vi "Text control_KM.vi"() -> ()   [LabVIEW 2016]
panel:
  in  "Panel Controls 2":T1={"Emergency Stop"=refnum, "TransGraph Max"=1e-05, "Text/Graph (text=false)"=FALSE, "TransGraph Min"=1e-11} {"TransGraph Min" format="%.2e"; "TransGraph Max" format="%.2e"}
  out "Currently running:":string
  in  "Lines left to run:":string
  in  "Standby":T2
  in  "Full Reset":bool
  in  "SMU4":cluster{"on/off":bool, "Voltage":dbl} {"Voltage" min=-100.0 max=100.0 format="%.2f"}
  in  "Source/Drain\nRange":u8(slide)=6 max=11 scale=0.0..11.0
  in  "Source/Drain\nRange mode":u16(ring) items=["Auto", "Limited", "Fixed"]
  in  "Gate Range":u8(slide)=6 max=11 scale=0.0..11.0
  in  "Gate Range\nmode":u16(ring) items=["Auto", "Limited", "Fixed"]
  in  "Gate":T3={"Gate Start"=0.0, "Gate Stop"=2.0, "Gate Step (linear only)"=1.0, "Gate Compliance"=0.0001, "Gate PComp"=0.0, "Range mode"=0, "Range"=6} {"Range" max=11 scale=0.0..11.0; "Range mode" items=["Auto", "Limited", "Fixed"]; "Gate PComp" format="%^.2e"; "Gate Compliance" format="%^.2e"; "Gate Step (linear only)" format="%^.4e"; "Gate Stop" format="%^.4e"; "Gate Start" format="%^.4e"}
  in  "Drain 2":T4={"Drain Start"=0.0, "Drain Stop"=2.0, "Drain Compliance"=0.0001, "Drain Step"=1.0, "Drain PComp"=0.0, "Range mode"=0, "Range"=6} {"Range" max=11 scale=0.0..11.0; "Range mode" items=["Auto", "Limited", "Fixed"]; "Drain PComp" format="%^.2e"; "Drain Step" format="%^.4e"; "Drain Compliance" format="%^.2e"; "Drain Stop" format="%^.4e"; "Drain Start" format="%^.4e"}
  in  "Timings 2":T5={"integration time"=0, "Short/Long integration time"=0.00064, "hold time (sec)"=0.0, "delay time (sec)"=0.0, "Step Time (0 disables)"=0.0, "sweep method"=0, "Pulse period"=0.005, "Base voltage"=0.0, "Pulse width"=0.0005} {"Pulse width" min=0.0005 max=0.1 step=0.0001 format="%.4f"; "Base voltage" format="%^.4e"; "Pulse period" min=0.005 max=1.0 step=0.0001 format="%.4f"; "sweep method" items=["Continuous", "Pulsed"]; "Step Time (0 disables)" format="%.2f"; "delay time (sec)" format="%.4f"; "hold time (sec)" format="%.4f"; "Short/Long integration time" format="%^.0e"; "integration time" scale=0.0..2.0}
  in  "Panel Controls":T6={"Emergency Stop"=refnum, "TransGraph Max"=1e-05, "Text/Graph (text=false)"=TRUE} {"TransGraph Max" format="%.2e"}
  in  "Interrupt run":bool
  in  "Drain: Compliance":dbl=0.001 format="%.8f"
  in  "Gate: Compliance":dbl=0.001 format="%.8f"
  out "Path":path
  in  "hold time /s":dbl format="%.2f"
  in  "delay time /s":dbl format="%.2f"
  in  "integration time":u32(slide)=1 max=2 step=1 scale=0.0..2.0
  in  "Integration time (short)":dbl=0.0019 min=8e-05 max=0.0019 step=8e-05 format="%^.0e"
  in  "Integration time (long)":dbl=0.32 min=0.04 max=2.0 step=0.02 format="%.2f"
  in  "Step delay /s":dbl format="%.2f"
  in  "Program":string="sample -60 -5 100 240\ntransfer d 10 -60 -1 -5 -60 -55"
  # "Syntax:\nsample Vg Vd NumSamples Time\nwait NumMilliseconds\nwait-min NumMinutes\ntransfer [s|d] VgStart VgStop VgStep VdStart VdStop VdStep\noutput [s|d] VgStart VgStop VgStep VdStart VdStop VdStep\nitime [s|m|l]\ngaterangemode [a|l|f]\ndrainrangemode [a|l|f]\nstandby [on l off]\nsample-fpp Vg Vd NumSamples Time\nresample-fpp Vg Vd\ntransfer-fpp [s|d] VgStart VgStop VgStep VdStart VdStop VdStep\noutput-fpp [s|d] VgStart VgStop VgStep VdStart VdStop VdStep"
  # "100 samples is approx 13s with medium integration"
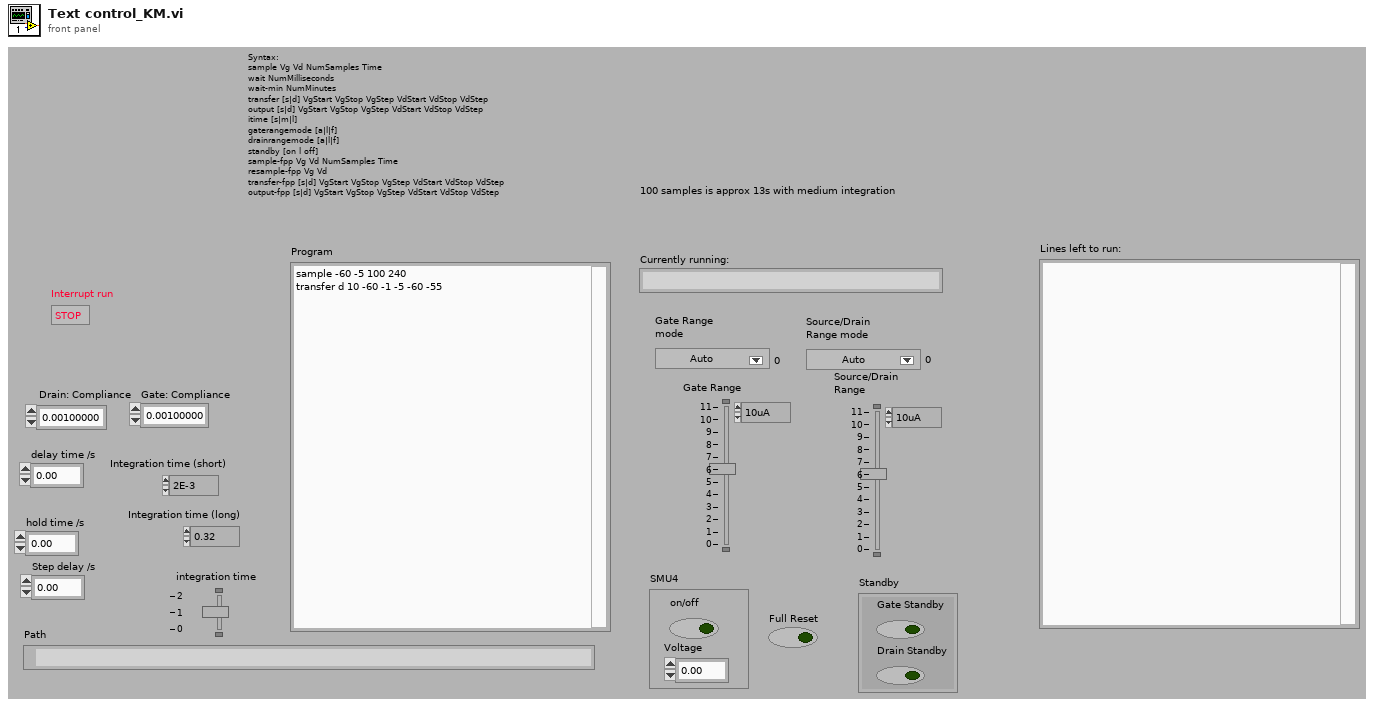
[diagram p1: front panel]
types:
  T1 = cluster{"Emergency Stop":refnum<vi>, "TransGraph Max":dbl, "Text/Graph (text=false)":bool, "TransGraph Min":dbl}
  T2 = cluster{"Gate Standby":bool, "Drain Standby":bool}
  T3 = cluster{"Gate Start":dbl, "Gate Stop":dbl, "Gate Step (linear only)":dbl, "Gate Compliance":dbl, "Gate PComp":dbl, "Range mode":u16, "Range":u8}
  T4 = cluster{"Drain Start":dbl, "Drain Stop":dbl, "Drain Compliance":dbl, "Drain Step":dbl, "Drain PComp":dbl, "Range mode":u16, "Range":u8}
  T5 = cluster{"integration time":u32, "Short/Long integration time":dbl, "hold time (sec)":dbl, "delay time (sec)":dbl, "Step Time (0 disables)":dbl, "sweep method":u16, "Pulse period":dbl, "Base voltage":dbl, "Pulse width":dbl}
  T6 = cluster{"Emergency Stop":refnum<vi>, "TransGraph Max":dbl, "Text/Graph (text=false)":bool}
  T7 = enum16{"open", "replace", "create", "open or create", "replace or create", "replace or create with confirmation"}
  T8 = cluster{"V2 Start":dbl, "V2 Step":dbl, "Number of points":i32}
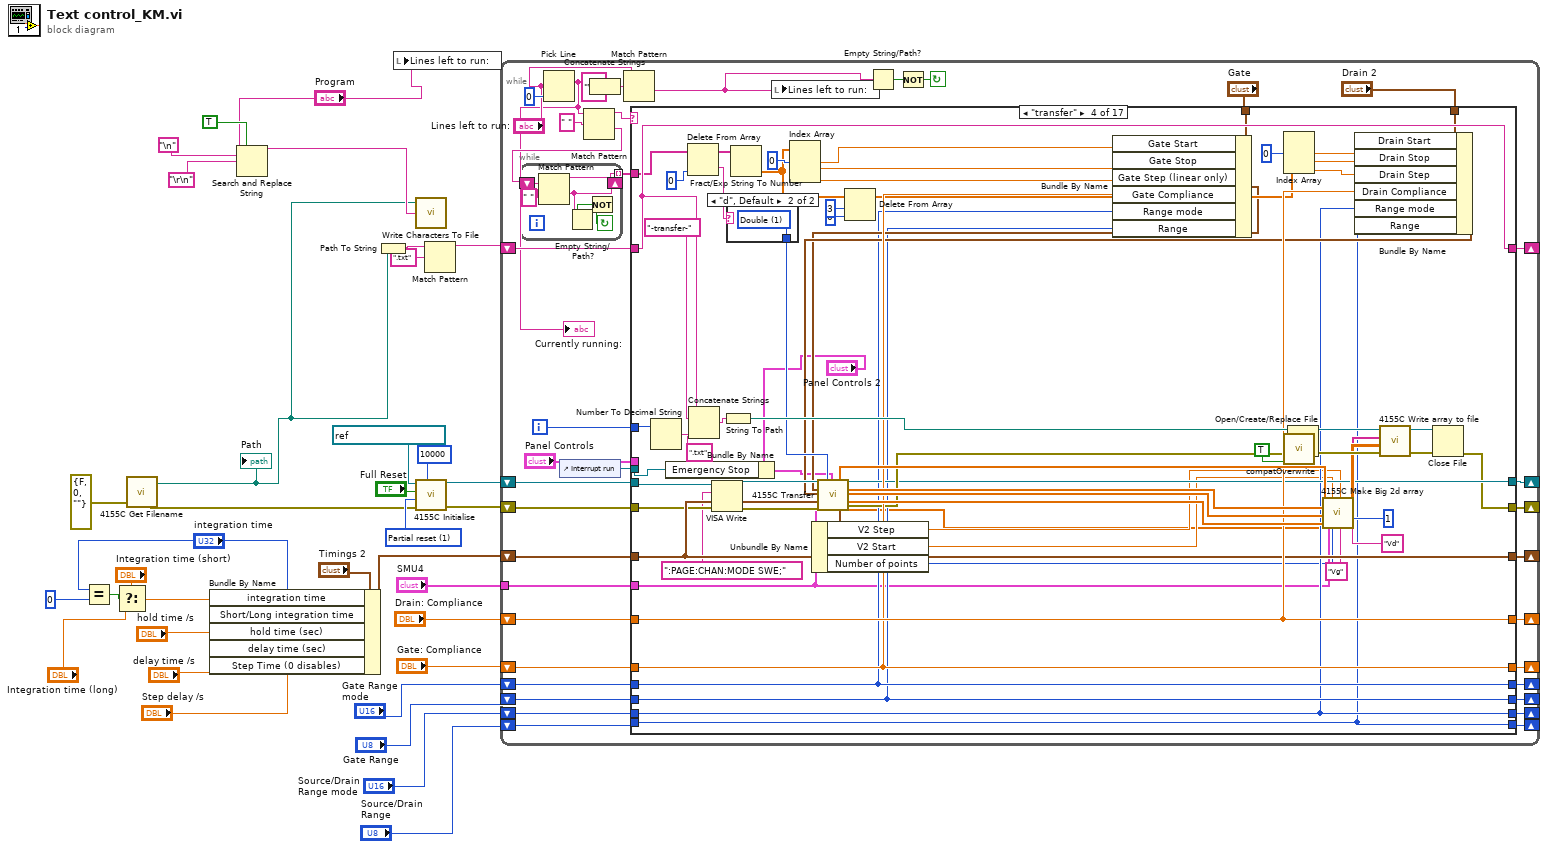
[diagram p0: block diagram]
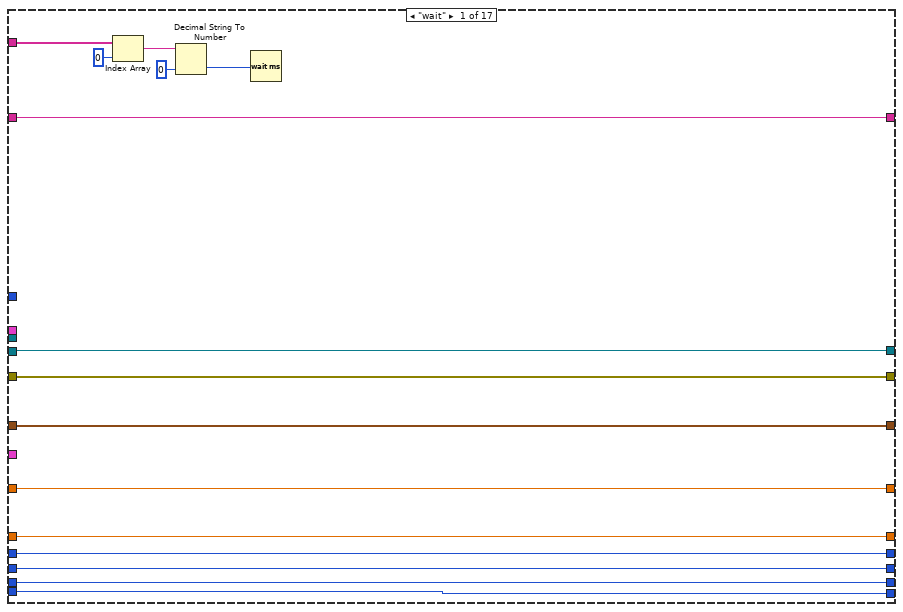
[diagram p2: hidden frame]
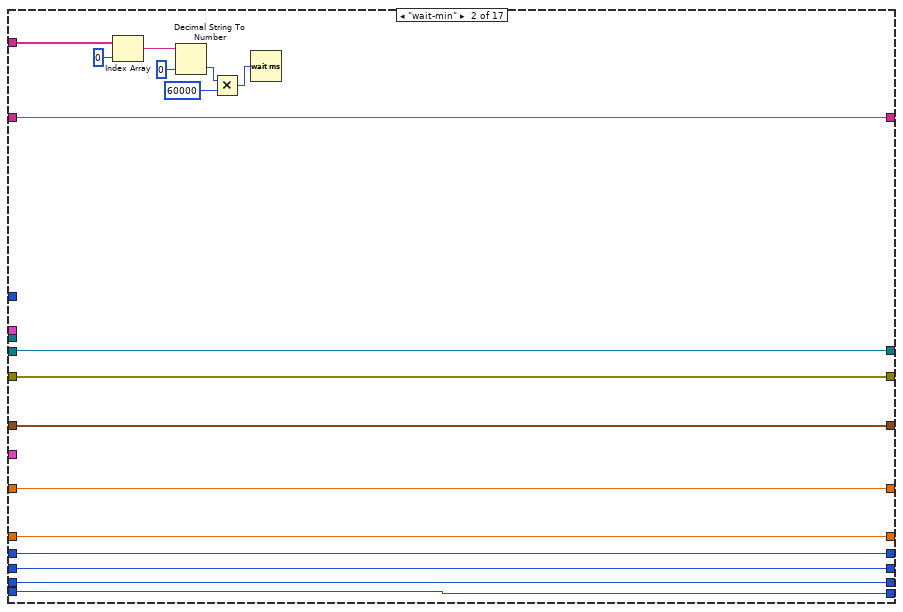
[diagram p3: hidden frame]
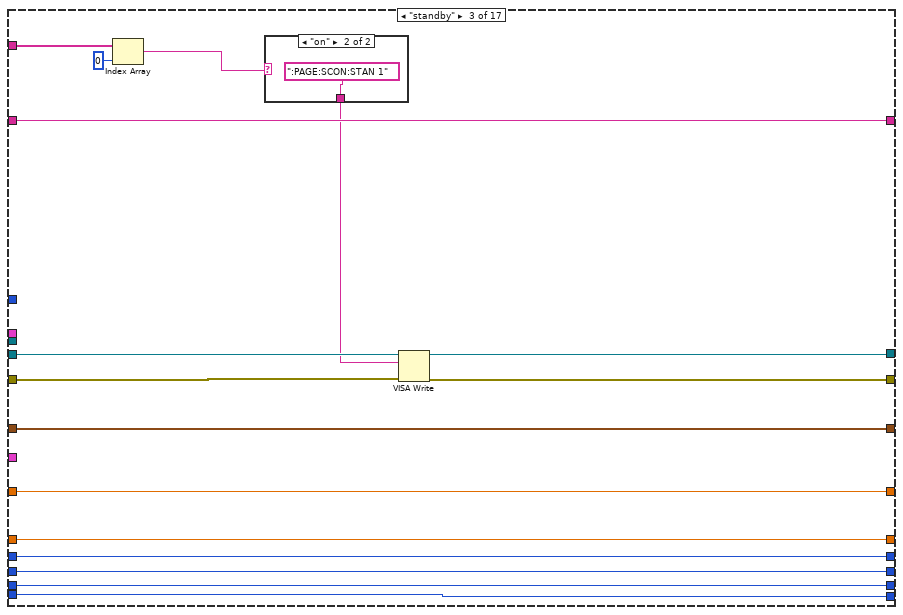
[diagram p4: hidden frame]
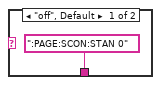
[diagram p5: hidden frame]
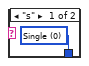
[diagram p6: hidden frame]
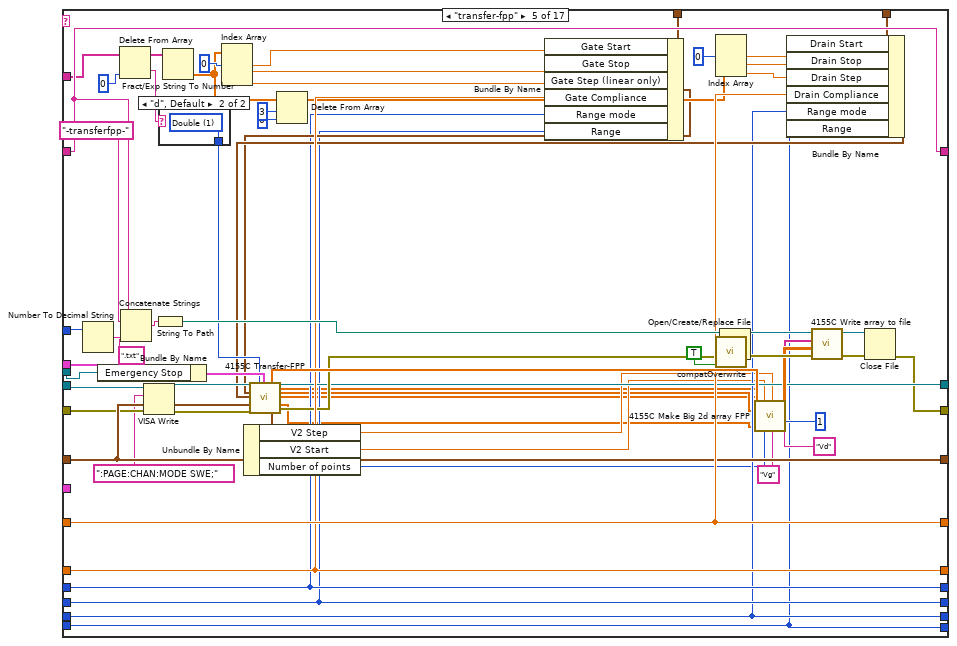
[diagram p7: hidden frame]
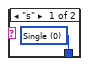
[diagram p8: hidden frame]
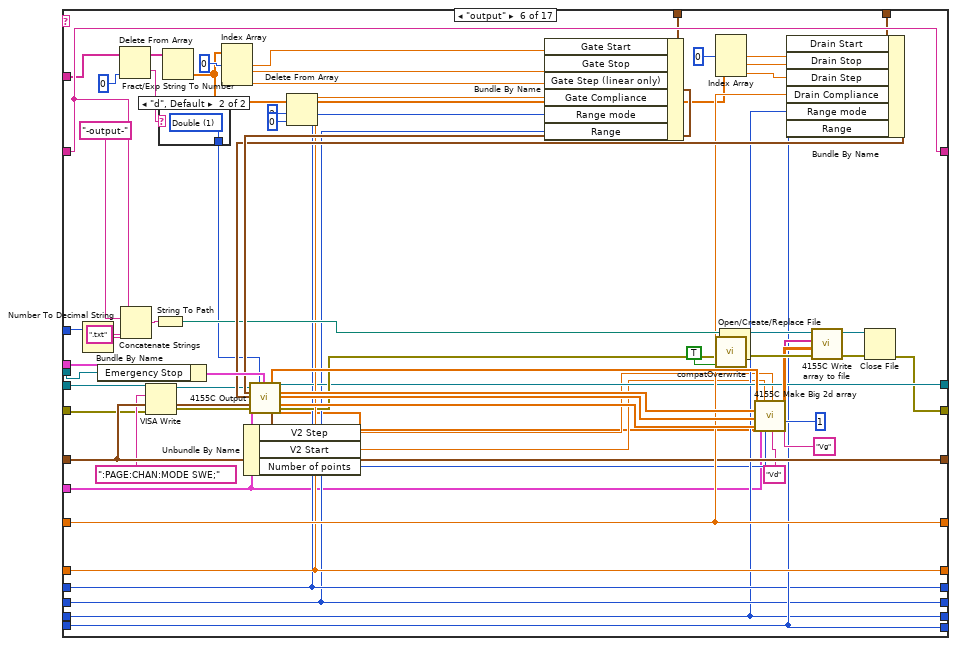
[diagram p9: hidden frame]
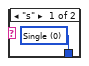
[diagram p10: hidden frame]
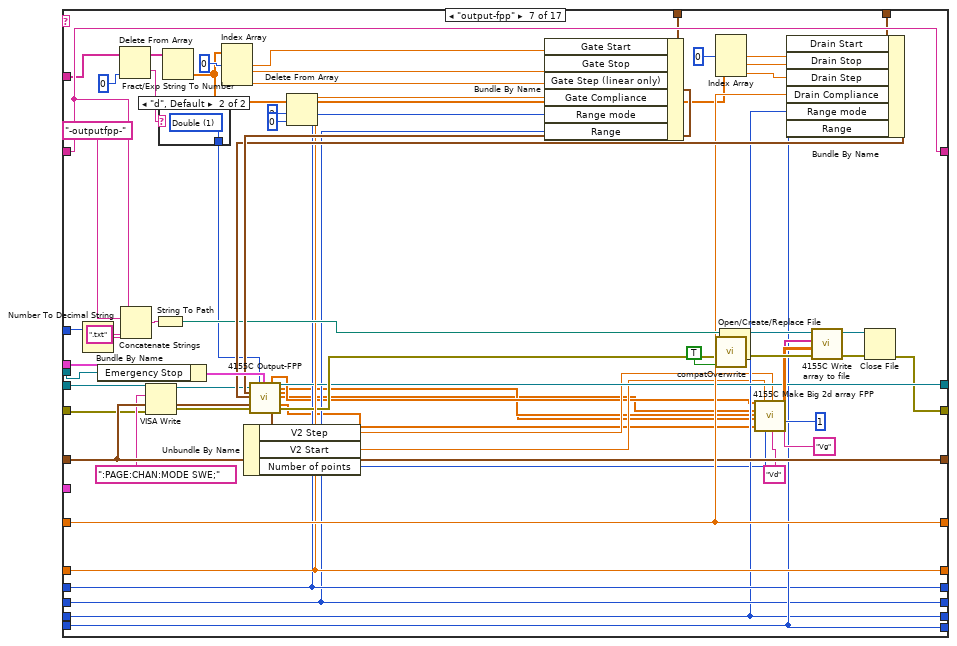
[diagram p11: hidden frame]
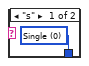
[diagram p12: hidden frame]
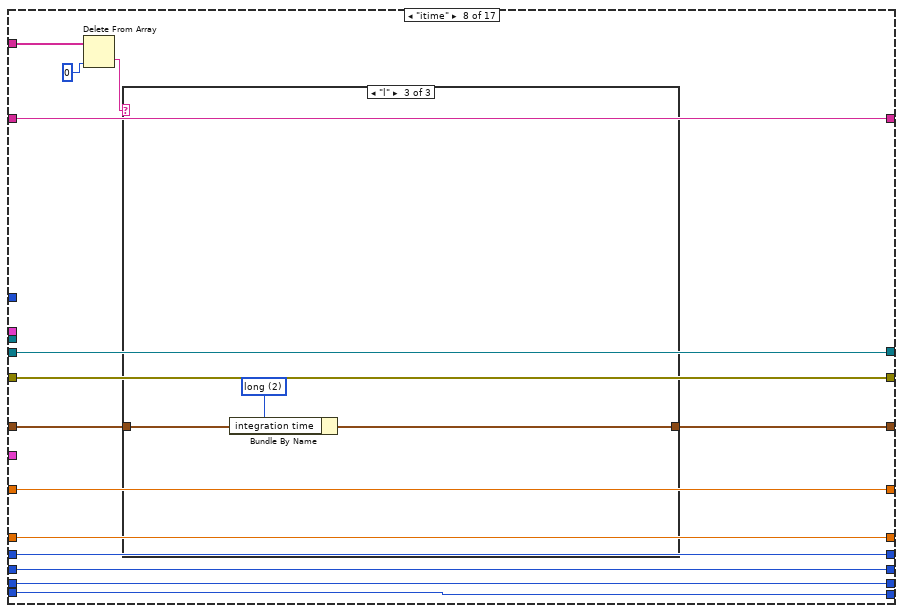
[diagram p13: hidden frame]
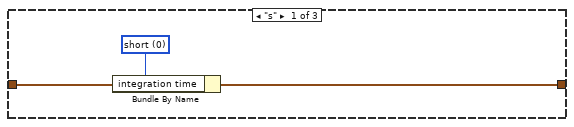
[diagram p14: hidden frame]
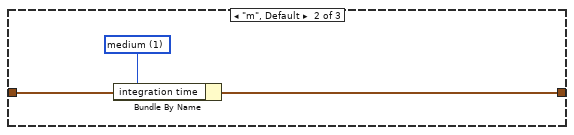
[diagram p15: hidden frame]
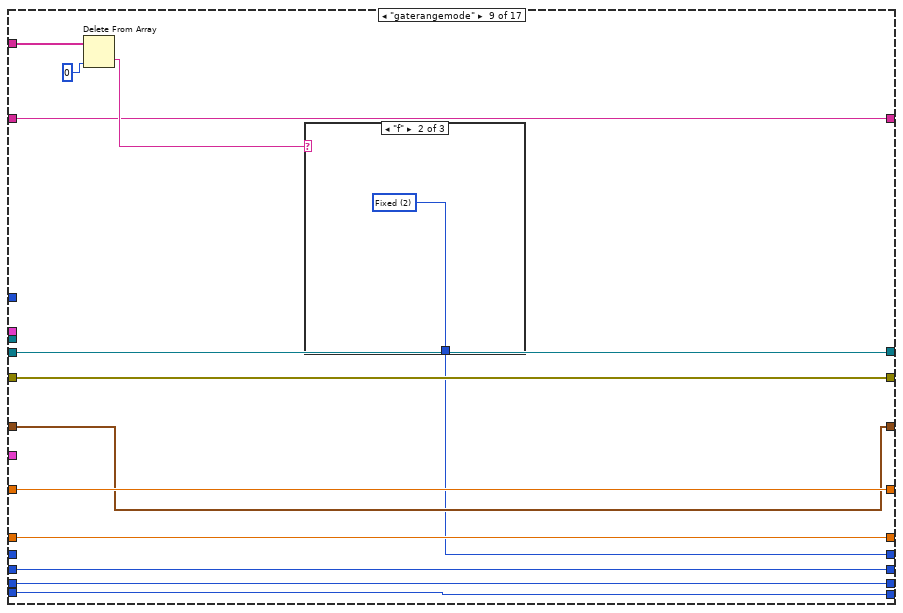
[diagram p16: hidden frame]
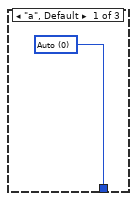
[diagram p17: hidden frame]
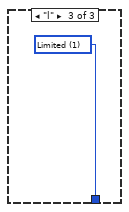
[diagram p18: hidden frame]
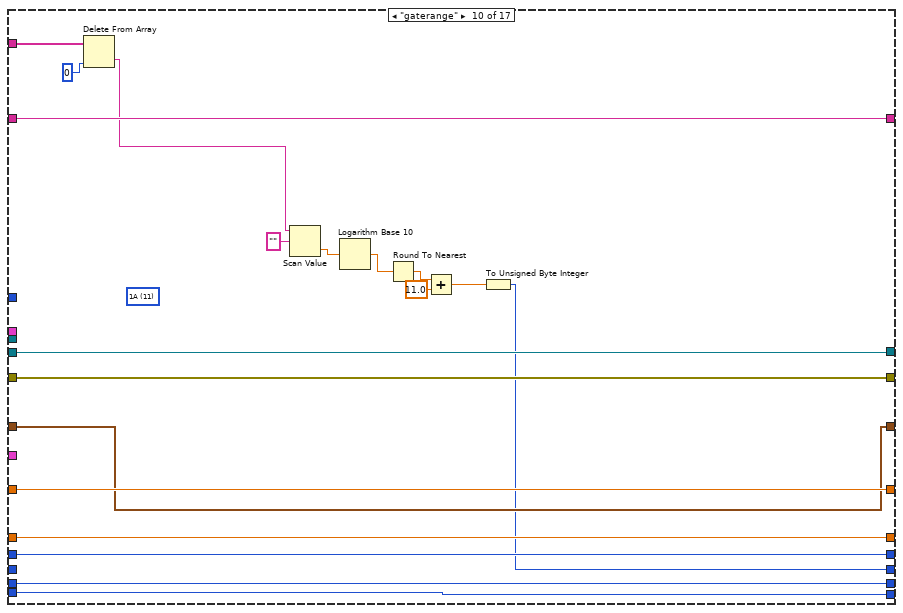
[diagram p19: hidden frame]
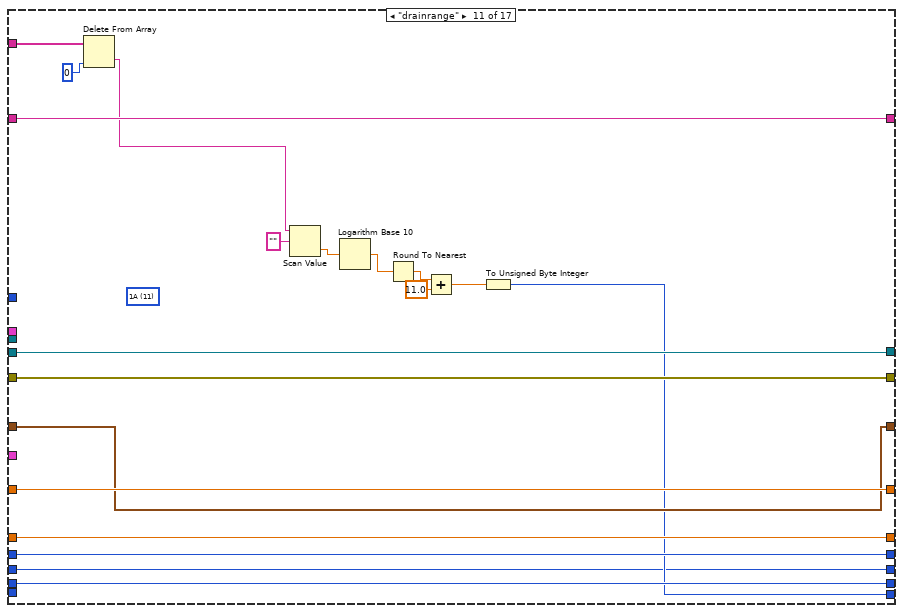
[diagram p20: hidden frame]
diagram:
  w26 = u16 1 items=["Reset All", "Partial reset"] ("Type of reset")
  n1 = Equal?(x="integration time", y=u32 0) -> (x = y?=w30:bool)
  n2 = Select(t="Integration time (short)", s=w30, f="Integration time (long)") -> (s? t:f=w34:dbl)
  n3 = call "4155C Get Filename.vi"("error in (no error)"=errorcluster {"status"=FALSE, "code"=0, "source"=""}) -> ("error out"=w21:errorcluster, "path"=w5:path)  [unwired: 2 in, 1 out]
  "Path" <- w5
  n4 = Bundle By Name(cluster="Timings 2", "integration time"="integration time", "Short/Long integration time"=w34, "hold time (sec)"="hold time /s", "delay time (sec)"="delay time /s", "Step Time (0 disables)"="Step delay /s") -> (w18:T5)
  n5 = Search and Replace String(replace all?=TRUE ("replace all? (F)"), input string="Program", search string="\n", replace string="\r\n") -> (result string=w8:string)  [unwired: 4 in, 3 out]
  n6 = Path To String(path=w5) -> (string=w4:string)
  n7 = local write "Lines left to run:"("Program") -> ()
  n8 = call <vilib>:"Write Characters To File.vi"("character string"=w8, "file path (dialog if empty)"=w5) -> ()  [unwired: 3 in, 1 out]
  n9 = call "4155C Initialise.vi"("VISA resource name in"=refnum<visa-resource-name> "GPIB0::14::INSTR", "Reset"="Full Reset", "Type of reset"=w26, "error in (no error)"=w21, "VISA Timeout Value"=u32 10000) -> ("VISA Resource Name out"=w20:refnum<visa-resource-name>, "error out"=w19:errorcluster)
  n10 = Match Pattern(string=w4, regular expression=".txt") -> (before substring=w3:string)  [unwired: 1 in, 3 out]
  n11 = while {
    tunnel: "SMU4" -> [w39]
    shift-left: "Source/Drain\nRange" -> [w44]
    shift-right: [w40] -> _
    shift-left: "Source/Drain\nRange mode" -> [w45]
    shift-right: [w41] -> _
    shift-left: "Gate Range" -> [w46]
    shift-right: [w42] -> _
    shift-left: "Gate Range\nmode" -> [w47]
    shift-right: [w43] -> _
    shift-left: "Gate: Compliance" -> [w59]
    shift-right: [w53] -> _
    shift-left: "Drain: Compliance" -> [w60]
    shift-right: [w54] -> _
    shift-left: w18 -> [w61]
    shift-right: [w55] -> _
    shift-left: w19 -> [w62]
    shift-right: [w56] -> _
    shift-left: w20 -> [w63]
    shift-right: [w57] -> _
    shift-left: w3 -> [w64]
    shift-right: [w52] -> _
    i -> [w58]
    stop <- w72 continue-if-true
    n12 = Pick Line(multi-line string="Lines left to run:", line index=0) -> (output string=w36:string)  [unwired: 1 in]
    "Currently running:" <- w36
    n13 = control-ref of="Interrupt run"() -> (w51:refnum<vi>)
    n14 = Match Pattern(string=w36, regular expression=" ") -> (before substring=w67:string, after substring=w66:string)  [unwired: 1 in, 2 out]
    n15 = while {
      tunnel: [w74] -> w65 mode=indexing
      shift-left: w66 -> [w76]
      shift-right: [w75] -> _
      stop <- w78 continue-if-true
      n16 = Match Pattern(string=w76, regular expression=" ") -> (before substring=w74:string, after substring=w75:string)  [unwired: 1 in, 2 out]
      n17 = Empty String/Path?(string/path=w75) -> (empty?=w79:bool)
      n18 = Not(x=w79) -> (.not. x?=w78:bool)
    }
    n19 = Concatenate Strings(w36, "\n" ("Substring")) -> (w70:string)
    n20 = Match Pattern(string="Lines left to run:", regular expression=w70) -> (after substring=w37:string)  [unwired: 1 in, 3 out]
    n21 = case shown="\"transfer\"" w67 {
      tunnel: w65 -> [w94 w111 w127 w172 w242 w306 w378 w415 w437 w460 w479 w491 _ _ w584 w653 w712]
      tunnel: w64 -> [w89 w107 w125 w180 w250 w314 w386 w404 w429 w453 w473 w484 w501 w539 w562 w647 w708]
      tunnel: w63 -> [w88 w106 w116 w150 w219 w282 w354 w405 w430 w454 w474 w485 w506 w542 w591 w660 w665]
      tunnel: w62 -> [w87 w105 w115 w149 w218 w279 w351 w406 w431 w455 w475 w486 w505 w511 w590 w659 w664]
      tunnel: w61 -> [w86 w104 w124 w176 w246 w310 w382 w414 w428 w452 w472 w483 w504 w535 w553 w646 w707]
      tunnel: w60 -> [w85 w103 w123 w178 w248 w312 w384 w413 w436 w459 w478 w490 w503 w520 w589 w658 w717]
      tunnel: w59 -> [w84 w102 w122 w177 w247 w311 w383 w412 w435 w458 w477 w489 w502 w521 w563 w648 w709]
      tunnel: w58 -> [_ _ _ w181 w251 w315 w387 _ _ _ _ _ _ w537 w588 w657 w716]
      tunnel: [w88 w106 w114 w174 w244 w308 w380 w405 w430 w454 w474 w485 w506 w542 w554 w599 w667] -> w57
      tunnel: [w87 w105 w113 w173 w243 w307 w379 w406 w431 w455 w475 w486 w505 w510 w564 w598 w666] -> w56
      tunnel: [w86 w104 w124 w176 w246 w310 w382 w407 w428 w452 w472 w483 w504 w535 w553 w646 w707] -> w55
      tunnel: [w85 w103 w123 w178 w248 w312 w384 w413 w436 w459 w478 w490 w503 w520 w589 w658 w717] -> w54
      tunnel: [w84 w102 w122 w177 w247 w311 w383 w412 w435 w458 w477 w489 w502 w521 w563 w648 w709] -> w53
      tunnel: [w89 w107 w125 w180 w250 w314 w386 w404 w429 w453 w473 w484 w501 w539 w562 w647 w708] -> w52
      tunnel: w51 -> [_ _ _ w189 w256 w323 w391 _ _ _ _ _ _ _ w559 w618 w683]
      tunnel: "Gate" -> [_ _ _ w159 w229 w293 w365 _ _ _ _ _ _ _ _ _ _]
      tunnel: "Drain 2" -> [_ _ _ w158 w228 w292 w364 _ _ _ _ _ _ _ _ _ _]
      tunnel: "Panel Controls" -> [_ _ _ _ w227 w291 w363 _ _ _ _ _ _ _ _ _ _]
      tunnel: w47 -> [w83 w101 w121 w143 w212 w277 w349 w411 _ w451 w471 w482 w500 w522 w549 w642 w703]
      tunnel: w46 -> [w82 w100 w120 w142 w211 w276 w348 w410 w434 _ w462 w488 w499 w523 w550 w643 w704]
      tunnel: w45 -> [w81 w99 w119 w141 w210 w275 w347 w409 w433 w457 w476 _ w498 w524 w551 w644 w705]
      tunnel: w44 -> [w80 w98 w118 w140 w209 w278 w350 w408 w432 w456 _ w487 w497 w525 w552 w645 w706]
      tunnel: [w83 w101 w121 w143 w212 w277 w349 w411 w427 w451 w471 w482 w500 w522 w549 w642 w703] -> w43
      tunnel: [w82 w100 w120 w142 w211 w276 w348 w410 w434 w443 w462 w488 w499 w523 w550 w643 w704] -> w42
      tunnel: [w81 w99 w119 w141 w210 w275 w347 w409 w433 w457 w476 w481 w498 w524 w551 w644 w705] -> w41
      tunnel: [w80 w98 w118 w140 w209 w278 w350 w408 w432 w456 w463 w487 w497 w525 w552 w645 w706] -> w40
      tunnel: w39 -> [_ _ _ w133 _ w269 _ _ _ _ _ _ _ _ _ _ _]
      frame "wait" {
        n22 = Index Array(array=w94, index=0 ("Index")) -> (element=w92:string)
        n23 = Decimal String To Number(string=w92, default (0L)=u32 0) -> (number=w91:u32)  [unwired: 1 in, 1 out]
        n24 = Wait (ms)(milliseconds to wait=w91) -> ()  [unwired: 1 out]
      }
      frame "wait-min" {
        n25 = Index Array(array=w111, index=0 ("Index")) -> (element=w109:string)
        n26 = Decimal String To Number(string=w109, default (0L)=u32 0) -> (number=w97:u32)  [unwired: 1 in, 1 out]
        n27 = Multiply(x=w97, y=u32 60000) -> (x*y=w96:u32)
        n28 = Wait (ms)(milliseconds to wait=w96) -> ()  [unwired: 1 out]
      }
      frame "standby" {
        n29 = Index Array(array=w127, index=0 ("Index")) -> (element=w117:string)
        n30 = case shown="\"on\"" w117 {
          tunnel: [":PAGE:SCON:STAN 0" ":PAGE:SCON:STAN 1"] -> w112
          frame "off", Default {
          }
          frame "on" {
          }
        }
        n31 = VISA Write(VISA resource name=w116, write buffer=w112, error in (no error)=w115) -> (VISA resource name out=w114:refnum<visa-resource-name>, error out=w113:errorcluster)  [unwired: 1 out]
      }
      frame "transfer" {
        n32 = Number To Decimal String(number=w181) -> (decimal integer string=w182:string)  [unwired: 1 in]
        n33 = Bundle By Name(cluster="Panel Controls 2", "Emergency Stop"=w189) -> (w131:T1)
        n34 = Delete From Array(array=w172, index=0 ("Index")) -> (deleted portion=w170:string, array with subset deleted=w169:string[])  [unwired: 1 in]
        n35 = Concatenate Strings(w180, "-transfer-" ("Substring"), w182, ".txt" ("Substring")) -> (w184:string)
        n36 = VISA Write(VISA resource name=w150, write buffer=":PAGE:CHAN:MODE SWE;" ("write buffer (\"\")"), error in (no error)=w149) -> (VISA resource name out=w147:refnum<visa-resource-name>, error out=w148:errorcluster)  [unwired: 1 out]
        n37 = String To Path(string=w184) -> (path=w179:path)
        n38 = case shown="\"d\", Default" w170 {
          tunnel: [w197 w198] -> w168
          frame "s" {
            w197 = u16 0 items=["Single", "Double"] ("sweep mode")
          }
          frame "d", Default {
            w198 = u16 1 items=["Single", "Double"] ("sweep mode")
          }
        }
        n39 = Fract/Exp String To Number(string=w169) -> (number=w154:dbl[])  [unwired: 3 in, 1 out]
        n40 = Index Array(array=w154, index #1=0 ("Index")) -> (element #1=w167:dbl, element #2=w166:dbl, element #3=w165:dbl)  [unwired: 2 in]
        n41 = Delete From Array(array=w154, length=3 ("Length"), index=0 ("Index")) -> (array with subset deleted=w152:dbl[])  [unwired: 1 out]
        n42 = Bundle By Name(cluster=w159, "Gate Start"=w167, "Gate Stop"=w166, "Gate Step (linear only)"=w165, "Gate Compliance"=w177, "Range mode"=w143, "Range"=w142) -> (w144:T3)
        n43 = Index Array(array=w152, index #1=0 ("Index")) -> (element #1=w162:dbl, element #2=w161:dbl, element #3=w160:dbl)  [unwired: 2 in]
        n44 = call <vilib>:"compatOverwrite.vi"("overwrite (F)"=TRUE) -> ("overwrite?"=w130:T7)
        n45 = Bundle By Name(cluster=w158, "Drain Start"=w162, "Drain Stop"=w161, "Drain Step"=w160, "Drain Compliance"=w178, "Range mode"=w141, "Range"=w140) -> (w145:T4)
        n46 = call "4155C Transfer.vi"("VISA resource name in"=w147, "Gate"=w144, "Drain"=w145, "Timings"=w176, "error in (no error)"=w148, "SMU4"=w133, "sweep mode"=w168, "Panel Controls"=w131) -> ("VG"=w185:dbl[], "Outparams"=w138:T8, "VISA Resource Name out"=w174:refnum<visa-resource-name>, "IS"=w188:dbl[], "ID"=w187:dbl[], "IG"=w186:dbl[], "error out"=w175:errorcluster, "SMU4"=w134:dbl[])  [unwired: 12 in]
        n47 = Unbundle By Name(w138) -> ("V2 Step"=w137:dbl, "V2 Start"=w136:dbl, "Number of points"=w135:i32)
        n48 = Open/Create/Replace File(file path (use dialog)=w179, error in=w175, operation (0:open)=w130) -> (refnum out=w194:refnum<file>, error out=w195:errorcluster)  [unwired: 3 in, 1 out]
        n49 = call "4155C Make Big 2d array.vi"("1D Var1"=w185, "1d IS"=w188, "1d ID"=w187, "1d IG"=w186, "1d SMU4"=w134, "SMU4"=w133, "VAR2 START"=w136, "Number of VAR2 steps"=w135, "VAR2 STEP"=w137, "VAR1 Name"="Vg", "Decimal places in header"=i8 1, "VAR2 Name"="Vd") -> ("Header array"=w190:string[], "Data array"=w191:dbl[][])  [unwired: 14 in]
        n50 = call "4155C Write array to file.vi"("Byte Stream File Refnum"=w194, "Header"=w190, "Data Array"=w191, "error in (no error)"=w195) -> ("dup refnum"=w192:refnum<file>, "error out"=w193:errorcluster)  [unwired: 1 in]
        n51 = Close File(refnum=w192, error in=w193) -> (error out=w173:errorcluster)  [unwired: 1 out]
      }
      frame "transfer-fpp" {
        n52 = Number To Decimal String(number=w251) -> (decimal integer string=w252:string)  [unwired: 1 in]
        n53 = Bundle By Name(cluster=w227, "Emergency Stop"=w256) -> (w264:T6)
        n54 = Delete From Array(array=w242, index=0 ("Index")) -> (deleted portion=w240:string, array with subset deleted=w239:string[])  [unwired: 1 in]
        n55 = Concatenate Strings(w250, "-transferfpp-" ("Substring"), w252, ".txt" ("Substring")) -> (w254:string)
        n56 = VISA Write(VISA resource name=w219, write buffer=":PAGE:CHAN:MODE SWE;" ("write buffer (\"\")"), error in (no error)=w218) -> (VISA resource name out=w216:refnum<visa-resource-name>, error out=w217:errorcluster)  [unwired: 1 out]
        n57 = String To Path(string=w254) -> (path=w249:path)
        n58 = case shown="\"d\", Default" w240 {
          tunnel: [w265 w266] -> w238
          frame "s" {
            w265 = u16 0 items=["Single", "Double"] ("sweep mode")
          }
          frame "d", Default {
            w266 = u16 1 items=["Single", "Double"] ("sweep mode")
          }
        }
        n59 = Fract/Exp String To Number(string=w239) -> (number=w223:dbl[])  [unwired: 3 in, 1 out]
        n60 = Index Array(array=w223, index #1=0 ("Index")) -> (element #1=w237:dbl, element #2=w236:dbl, element #3=w235:dbl)  [unwired: 2 in]
        n61 = Delete From Array(array=w223, length=3 ("Length"), index=0 ("Index")) -> (array with subset deleted=w221:dbl[])  [unwired: 1 out]
        n62 = Bundle By Name(cluster=w229, "Gate Start"=w237, "Gate Stop"=w236, "Gate Step (linear only)"=w235, "Gate Compliance"=w247, "Range mode"=w212, "Range"=w211) -> (w213:T3)
        n63 = Index Array(array=w221, index #1=0 ("Index")) -> (element #1=w232:dbl, element #2=w231:dbl, element #3=w230:dbl)  [unwired: 2 in]
        n64 = call <vilib>:"compatOverwrite.vi"("overwrite (F)"=TRUE) -> ("overwrite?"=w199:T7)
        n65 = Bundle By Name(cluster=w228, "Drain Start"=w232, "Drain Stop"=w231, "Drain Step"=w230, "Drain Compliance"=w248, "Range mode"=w210, "Range"=w209) -> (w214:T4)
        n66 = call "4155C Transfer-FPP.vi"("VISA resource name in"=w216, "Gate"=w213, "Drain"=w214, "Timings"=w246, "error in (no error)"=w217, "sweep mode"=w238, "Panel Controls"=w264) -> ("VG"=w255:dbl[], "Outparams"=w207:T8, "VISA Resource Name out"=w244:refnum<visa-resource-name>, "Vprobe2"=w203:dbl[], "ID"=w202:dbl[], "IG"=w201:dbl[], "Vprobe1"=w200:dbl[], "error out"=w245:errorcluster)  [unwired: 13 in]
        n67 = Unbundle By Name(w207) -> ("V2 Step"=w206:dbl, "V2 Start"=w205:dbl, "Number of points"=w204:i32)
        n68 = Open/Create/Replace File(file path (use dialog)=w249, error in=w245, operation (0:open)=w199) -> (refnum out=w261:refnum<file>, error out=w262:errorcluster)  [unwired: 3 in, 1 out]
        n69 = call "4155C Make Big 2d array FPP.vi"("1D Var1"=w255, "1d ID"=w202, "1d Vp2"=w203, "1d IG"=w201, "1d Vp1"=w200, "VAR2 START"=w205, "Number of VAR2 steps"=w204, "VAR2 STEP"=w206, "VAR1 Name"="Vg", "Decimal places in header"=i8 1, "VAR2 Name"="Vd") -> ("Header array"=w257:string[], "Data array"=w258:dbl[][])  [unwired: 15 in]
        n70 = call "4155C Write array to file.vi"("Byte Stream File Refnum"=w261, "Header"=w257, "Data Array"=w258, "error in (no error)"=w262) -> ("dup refnum"=w259:refnum<file>, "error out"=w260:errorcluster)  [unwired: 1 in]
        n71 = Close File(refnum=w259, error in=w260) -> (error out=w243:errorcluster)  [unwired: 1 out]
      }
      frame "output" {
        n72 = Number To Decimal String(number=w315) -> (decimal integer string=w316:string)  [unwired: 1 in]
        n73 = Bundle By Name(cluster=w291, "Emergency Stop"=w323) -> (w333:T6)
        n74 = Delete From Array(array=w306, index=0 ("Index")) -> (deleted portion=w304:string, array with subset deleted=w303:string[])  [unwired: 1 in]
        n75 = Concatenate Strings(w314, "-output-" ("Substring"), w316, ".txt" ("Substring")) -> (w318:string)
        n76 = VISA Write(VISA resource name=w282, write buffer=":PAGE:CHAN:MODE SWE;" ("write buffer (\"\")"), error in (no error)=w279) -> (VISA resource name out=w281:refnum<visa-resource-name>, error out=w280:errorcluster)  [unwired: 1 out]
        n77 = String To Path(string=w318) -> (path=w313:path)
        n78 = case shown="\"d\", Default" w304 {
          tunnel: [w334 w335] -> w302
          frame "s" {
            w334 = u16 0 items=["Single", "Double"] ("sweep mode")
          }
          frame "d", Default {
            w335 = u16 1 items=["Single", "Double"] ("sweep mode")
          }
        }
        n79 = Fract/Exp String To Number(string=w303) -> (number=w285:dbl[])  [unwired: 3 in, 1 out]
        n80 = Index Array(array=w285, index #1=0 ("Index")) -> (element #1=w301:dbl, element #2=w300:dbl, element #3=w299:dbl)  [unwired: 2 in]
        n81 = Delete From Array(array=w285, length=3 ("Length"), index=0 ("Index")) -> (array with subset deleted=w284:dbl[])  [unwired: 1 out]
        n82 = Bundle By Name(cluster=w293, "Gate Start"=w301, "Gate Stop"=w300, "Gate Step (linear only)"=w299, "Gate Compliance"=w311, "Range mode"=w277, "Range"=w276) -> (w332:T3)
        n83 = Index Array(array=w284, index #1=0 ("Index")) -> (element #1=w296:dbl, element #2=w295:dbl, element #3=w294:dbl)  [unwired: 2 in]
        n84 = call <vilib>:"compatOverwrite.vi"("overwrite (F)"=TRUE) -> ("overwrite?"=w267:T7)
        n85 = Bundle By Name(cluster=w292, "Drain Start"=w296, "Drain Stop"=w295, "Drain Step"=w294, "Drain Compliance"=w312, "Range mode"=w275, "Range"=w278) -> (w331:T4)
        n86 = call "4155C Output.vi"("VISA resource name in"=w281, "Gate"=w332, "Drain"=w331, "Timings"=w310, "error in (no error)"=w280, "SMU4"=w269, "sweep mode"=w302, "Panel controls"=w333) -> ("VD"=w319:dbl[], "Outparams"=w272:T8, "VISA Resource Name out"=w308:refnum<visa-resource-name>, "IS"=w322:dbl[], "ID"=w321:dbl[], "IG"=w320:dbl[], "error out"=w309:errorcluster, "SMU4"=w268:dbl[])  [unwired: 12 in]
        n87 = Unbundle By Name(w272) -> ("V2 Step"=w273:dbl, "V2 Start"=w271:dbl, "Number of points"=w270:i32)
        n88 = Open/Create/Replace File(file path (use dialog)=w313, error in=w309, operation (0:open)=w267) -> (refnum out=w328:refnum<file>, error out=w329:errorcluster)  [unwired: 3 in, 1 out]
        n89 = call "4155C Make Big 2d array.vi"("1D Var1"=w319, "1d IS"=w322, "1d ID"=w321, "1d IG"=w320, "1d SMU4"=w268, "SMU4"=w269, "VAR2 START"=w271, "Number of VAR2 steps"=w270, "VAR2 STEP"=w273, "VAR1 Name"="Vd", "Decimal places in header"=i8 1, "VAR2 Name"="Vg") -> ("Header array"=w324:string[], "Data array"=w325:dbl[][])  [unwired: 14 in]
        n90 = call "4155C Write array to file.vi"("Byte Stream File Refnum"=w328, "Header"=w324, "Data Array"=w325, "error in (no error)"=w329) -> ("dup refnum"=w326:refnum<file>, "error out"=w327:errorcluster)  [unwired: 1 in]
        n91 = Close File(refnum=w326, error in=w327) -> (error out=w307:errorcluster)  [unwired: 1 out]
      }
      frame "output-fpp" {
        n92 = Number To Decimal String(number=w387) -> (decimal integer string=w388:string)  [unwired: 1 in]
        n93 = Bundle By Name(cluster=w363, "Emergency Stop"=w391) -> (w401:T6)
        n94 = Delete From Array(array=w378, index=0 ("Index")) -> (deleted portion=w376:string, array with subset deleted=w375:string[])  [unwired: 1 in]
        n95 = Concatenate Strings(w386, "-outputfpp-" ("Substring"), w388, ".txt" ("Substring")) -> (w390:string)
        n96 = VISA Write(VISA resource name=w354, write buffer=":PAGE:CHAN:MODE SWE;" ("write buffer (\"\")"), error in (no error)=w351) -> (VISA resource name out=w353:refnum<visa-resource-name>, error out=w352:errorcluster)  [unwired: 1 out]
        n97 = String To Path(string=w390) -> (path=w385:path)
        n98 = case shown="\"d\", Default" w376 {
          tunnel: [w402 w403] -> w374
          frame "s" {
            w402 = u16 0 items=["Single", "Double"] ("sweep mode")
          }
          frame "d", Default {
            w403 = u16 1 items=["Single", "Double"] ("sweep mode")
          }
        }
        n99 = Fract/Exp String To Number(string=w375) -> (number=w357:dbl[])  [unwired: 3 in, 1 out]
        n100 = Index Array(array=w357, index #1=0 ("Index")) -> (element #1=w373:dbl, element #2=w372:dbl, element #3=w371:dbl)  [unwired: 2 in]
        n101 = Delete From Array(array=w357, length=3 ("Length"), index=0 ("Index")) -> (array with subset deleted=w356:dbl[])  [unwired: 1 out]
        n102 = Bundle By Name(cluster=w365, "Gate Start"=w373, "Gate Stop"=w372, "Gate Step (linear only)"=w371, "Gate Compliance"=w383, "Range mode"=w349, "Range"=w348) -> (w400:T3)
        n103 = Index Array(array=w356, index #1=0 ("Index")) -> (element #1=w368:dbl, element #2=w367:dbl, element #3=w366:dbl)  [unwired: 2 in]
        n104 = call <vilib>:"compatOverwrite.vi"("overwrite (F)"=TRUE) -> ("overwrite?"=w336:T7)
        n105 = Bundle By Name(cluster=w364, "Drain Start"=w368, "Drain Stop"=w367, "Drain Step"=w366, "Drain Compliance"=w384, "Range mode"=w347, "Range"=w350) -> (w399:T4)
        n106 = call "4155C Output-FPP.vi"("VISA resource name in"=w353, "Gate"=w400, "Drain"=w399, "Timings"=w382, "error in (no error)"=w352, "sweep mode"=w374, "Panel controls"=w401) -> ("VD"=w341:dbl[], "Outparams"=w344:T8, "VISA Resource Name out"=w380:refnum<visa-resource-name>, "Vprobe2"=w340:dbl[], "ID"=w339:dbl[], "IG"=w338:dbl[], "Vprobe1"=w337:dbl[], "error out"=w381:errorcluster)  [unwired: 13 in]
        n107 = Unbundle By Name(w344) -> ("V2 Step"=w345:dbl, "V2 Start"=w343:dbl, "Number of points"=w342:i32)
        n108 = Open/Create/Replace File(file path (use dialog)=w385, error in=w381, operation (0:open)=w336) -> (refnum out=w396:refnum<file>, error out=w397:errorcluster)  [unwired: 3 in, 1 out]
        n109 = call "4155C Make Big 2d array FPP.vi"("1D Var1"=w341, "1d ID"=w339, "1d Vp2"=w340, "1d IG"=w338, "1d Vp1"=w337, "VAR2 START"=w343, "Number of VAR2 steps"=w342, "VAR2 STEP"=w345, "VAR1 Name"="Vd", "Decimal places in header"=i8 1, "VAR2 Name"="Vg") -> ("Header array"=w392:string[], "Data array"=w393:dbl[][])  [unwired: 15 in]
        n110 = call "4155C Write array to file.vi"("Byte Stream File Refnum"=w396, "Header"=w392, "Data Array"=w393, "error in (no error)"=w397) -> ("dup refnum"=w394:refnum<file>, "error out"=w395:errorcluster)  [unwired: 1 in]
        n111 = Close File(refnum=w394, error in=w395) -> (error out=w379:errorcluster)  [unwired: 1 out]
      }
      frame "itime" {
        n112 = Delete From Array(array=w415, index=0 ("Index")) -> (deleted portion=w416:string)  [unwired: 1 in, 1 out]
        n113 = case shown="\"l\"" w416 {
          tunnel: w414 -> [w420 w422 w425]
          tunnel: [w419 w421 w424] -> w407
          frame "s" {
            w418 = u32 0 items=["short  ", "medium  ", "long  "] ("integration time 2")
            n114 = Bundle By Name(cluster=w420, "integration time"=w418) -> (w419:T5)
          }
          frame "m", Default {
            w423 = u32 1 items=["short  ", "medium  ", "long  "] ("integration time 2")
            n115 = Bundle By Name(cluster=w422, "integration time"=w423) -> (w421:T5)
          }
          frame "l" {
            w426 = u32 2 items=["short  ", "medium  ", "long  "] ("integration time 2")
            n116 = Bundle By Name(cluster=w425, "integration time"=w426) -> (w424:T5)
          }
        }
      }
      frame "gaterangemode" {
        n117 = Delete From Array(array=w437, index=0 ("Index")) -> (deleted portion=w438:string)  [unwired: 1 in, 1 out]
        n118 = case shown="\"f\"" w438 {
          tunnel: [w440 w441 w442] -> w427
          frame "a", Default {
            w440 = u16 0 items=["Auto", "Limited", "Fixed"] ("Gate Range\nmode 2")
          }
          frame "f" {
            w441 = u16 2 items=["Auto", "Limited", "Fixed"] ("Gate Range\nmode 2")
          }
          frame "l" {
            w442 = u16 1 items=["Auto", "Limited", "Fixed"] ("Gate Range\nmode 2")
          }
        }
      }
      frame "gaterange" {
        (unwired) u8 11 items=["10fA  ", "100fA  ", "1nA  ", "10nA", "100nA", "1uA", "10uA", "100uA", "1mA", "10mA", "100mA", "1A"] ("Gate Range 2")
        n119 = Delete From Array(array=w460, index=0 ("Index")) -> (deleted portion=w450:string)  [unwired: 1 in, 1 out]
        n120 = Scan Value(string=w450, format string="") -> (value=w448:dbl)  [unwired: 1 in, 1 out]
        n121 = Logarithm Base 10(1:w448) -> (0:w447:dbl)
        n122 = Round To Nearest(number=w447) -> (nearest integer value=w446:dbl)
        n123 = Add(x=w446, y=11.0) -> (x+y=w444:dbl)
        n124 = To Unsigned Byte Integer(number=w444) -> (unsigned 8bit integer=w443:u8)
      }
      frame "drainrange" {
        (unwired) u8 11 items=["10fA  ", "100fA  ", "1nA  ", "10nA", "100nA", "1uA", "10uA", "100uA", "1mA", "10mA", "100mA", "1A"] ("Gate Range 2")
        n125 = Delete From Array(array=w479, index=0 ("Index")) -> (deleted portion=w470:string)  [unwired: 1 in, 1 out]
        n126 = Scan Value(string=w470, format string="") -> (value=w468:dbl)  [unwired: 1 in, 1 out]
        n127 = Logarithm Base 10(1:w468) -> (0:w467:dbl)
        n128 = Round To Nearest(number=w467) -> (nearest integer value=w466:dbl)
        n129 = Add(x=w466, y=11.0) -> (x+y=w464:dbl)
        n130 = To Unsigned Byte Integer(number=w464) -> (unsigned 8bit integer=w463:u8)
      }
      frame "drainrangemode" {
        n131 = Delete From Array(array=w491, index=0 ("Index")) -> (deleted portion=w492:string)  [unwired: 1 in, 1 out]
        n132 = case shown="\"f\"" w492 {
          tunnel: [w494 w495 w496] -> w481
          frame "a", Default {
            w494 = u16 0 items=["Auto", "Limited", "Fixed"] ("Gate Range\nmode 2")
          }
          frame "f" {
            w495 = u16 2 items=["Auto", "Limited", "Fixed"] ("Gate Range\nmode 2")
          }
          frame "l" {
            w496 = u16 1 items=["Auto", "Limited", "Fixed"] ("Gate Range\nmode 2")
          }
        }
      }
      frame "Error", Default {
      }
      frame "logfile" {
        n133 = Number To Decimal String(number=w537) -> (decimal integer string=w541:string)  [unwired: 1 in]
        n134 = Concatenate Strings(w539, "logfile" ("Substring"), w541, ".txt" ("Substring")) -> (w536:string)
        n135 = String To Path(string=w536) -> (path=w509:path)
        n136 = Unbundle(w535) -> ("integration time"=w534:u32, "Short/Long integration time"=w533:dbl, "hold time (sec)"=w532:dbl, "delay time (sec)"=w531:dbl, "Step Time (0 disables)"=w530:dbl, "sweep method"=w529:u16, "Pulse period"=w528:dbl, "Base voltage"=w527:dbl, "Pulse width"=w526:dbl)
        n137 = Build Array(w534, w533, w532, w531, w530, w529, w528, w527, w526, w520, w521, w522, w523, w524, w525) -> (w513:dbl[])
        n138 = Insert Into Array(array=dbl[][] [] ("Input Array"), new element=w513) -> (w512:dbl[][])  [unwired: 2 in]
        n139 = call <vilib>:"compatOverwrite.vi"("overwrite (F)"=TRUE) -> ("overwrite?"=w507:T7)
        n140 = Open/Create/Replace File(file path (use dialog)=w509, error in=w511, operation (0:open)=w507) -> (refnum out=w517:refnum<file>, error out=w516:errorcluster)  [unwired: 3 in, 1 out]
        n141 = call "4155C Write array to file.vi"("Byte Stream File Refnum"=w517, "Header"=string[] ["Int Time", "Short/Long Itime", "Hold time", "Delay time", "Step time", "Sweep method", "Pulse period", "Base Voltage", "Pulse width", "Drain compliance", "Gate compliance", "Gate range mode", "Gate range", "S/D range mode", "S/D range"], "Data Array"=w512, "error in (no error)"=w516) -> ("dup refnum"=w519:refnum<file>, "error out"=w518:errorcluster)  [unwired: 1 in]
        n142 = Close File(refnum=w519, error in=w518) -> (error out=w510:errorcluster)  [unwired: 1 out]
      }
      frame "sample" {
        n143 = Number To Decimal String(number=w588) -> (decimal integer string=w587:string)  [unwired: 1 in]
        n144 = Fract/Exp String To Number(string=w584) -> (number=w548:dbl[])  [unwired: 3 in, 1 out]
        n145 = Concatenate Strings(w562, "-sample-" ("Substring"), w587, ".txt" ("Substring")) -> (w585:string)
        n146 = String To Path(string=w585) -> (path=w566:path)
        n147 = Index Array(array=w548, index=0 ("Index")) -> (element=w582:dbl)
        n148 = Index Array(array=w548, index=1 ("Index")) -> (element=w579:dbl)
        n149 = Index Array(array=w548, index=2 ("Index")) -> (element=w578:dbl)
        n150 = Index Array(array=w548, index=3 ("Index")) -> (element=w546:dbl)
        n151 = call "4155C Config Sampling Measurements.vi"("Sample time"=w546, "Display on/off"=TRUE, "Timings"=w553, "Num Points"=w578, "error in (no error)"=w590, "Drain Compliance"=w589, "Gate Compliance"=w563, "VISA session"=w591) -> ("error out"=w592:errorcluster, "dup VISA resource name"=w593:refnum<visa-resource-name>)  [unwired: 2 in]
        n152 = call "4155C Take Sample.vi"("Emergency Stop"=w559, "error in (no error)"=w592, "Vd"=w579, "Vg"=w582, "VISA resource name in"=w593) -> ("error out"=w557:errorcluster, "Id"=w595:dbl[], "Ig"=w568:dbl[], "VISA Resource Name out"=w555:refnum<visa-resource-name>, "Is"=w594:dbl[], "Time"=w572:dbl[])  [unwired: 1 in]
        n153 = Insert Into Array(array=dbl[][] [] ("Input Array"), new element=w572) -> (w571:dbl[][])  [unwired: 2 in]
        n154 = Insert Into Array(array=w571, new element=w568) -> (w570:dbl[][])  [unwired: 2 in]
        n155 = Insert Into Array(array=w570, new element=w595) -> (w569:dbl[][])  [unwired: 2 in]
        n156 = VISA Write(VISA resource name=w555, write buffer=":DISP ON" ("write buffer (\"\")"), error in (no error)=w557) -> (VISA resource name out=w554:refnum<visa-resource-name>, error out=w556:errorcluster)  [unwired: 1 out]
        n157 = Insert Into Array(array=w569, new element=w594) -> (w561:dbl[][])  [unwired: 2 in]
        n158 = Transpose 2D Array(2D array=w561) -> (transposed array=w560:dbl[][])
        n159 = call <vilib>:"compatOverwrite.vi"("overwrite (F)"=TRUE) -> ("overwrite?"=w543:T7)
        n160 = Open/Create/Replace File(file path (use dialog)=w566, error in=w556, operation (0:open)=w543) -> (refnum out=w575:refnum<file>, error out=w574:errorcluster)  [unwired: 3 in, 1 out]
        n161 = call "4155C Write array to file.vi"("Byte Stream File Refnum"=w575, "Header"=string[] ["Time /s", "Ig /A", "Id /A", "Is /A"], "Data Array"=w560, "error in (no error)"=w574) -> ("dup refnum"=w577:refnum<file>, "error out"=w576:errorcluster)  [unwired: 1 in]
        n162 = Close File(refnum=w577, error in=w576) -> (error out=w564:errorcluster)  [unwired: 1 out]
      }
      frame "sample-fpp" {
        w603 = string[] ["Time /s", "Id VgVd /A", "Ig VgVd /A", "Vp1 VgVd /V", "Vp2 VgVd /V"] ("Header")
        w607 = "%d" ("format string")
        n163 = Number To Decimal String(number=w657) -> (decimal integer string=w656:string)  [unwired: 1 in]
        n164 = Fract/Exp String To Number(string=w653) -> (number=w641:dbl[])  [unwired: 3 in, 1 out]
        n165 = Concatenate Strings(w647, "-samplefpp-" ("Substring"), w656, ".txt" ("Substring")) -> (w654:string)
        n166 = String To Path(string=w654) -> (path=w615:path)
        n167 = Index Array(array=w641, index=0 ("Index")) -> (element=w601:dbl)
        n168 = Index Array(array=w641, index=1 ("Index")) -> (element=w600:dbl)
        n169 = Index Array(array=w641, index=2 ("Index")) -> (element=w649:dbl)
        n170 = Index Array(array=w641, index=3 ("Index")) -> (element=w639:dbl)
        n171 = call "4155C Config Sampling Measurements FPP.vi"("VISA session"=w660, "Num Points"=w649, "Vg"=w601, "Display on/off"=TRUE, "Gate Compliance"=w648, "Drain Compliance"=w658, "Standby"="Standby", "error in (no error)"=w659, "Timings"=w646, "Vd"=w600, "Sample time"=w639) -> ("dup VISA resource name"=w617:refnum<visa-resource-name>, "error out"=w616:errorcluster)  [unwired: 3 in]
        n172 = Number To Decimal String(number=w601) -> (decimal integer string=w627:string)  [unwired: 1 in]
        n173 = call "4155C Take Sample FPP.vi"("VISA resource name in"=w617, "error in (no error)"=w616, "Emergency Stop"=w618) -> ("Time"=w622:dbl[], "Vp1"=w632:dbl[], "VISA Resource Name out"=w599:refnum<visa-resource-name>, "Ig"=w620:dbl[], "Id"=w621:dbl[], "Vp2"=w630:dbl[], "error out"=w619:errorcluster)  [unwired: 10 in]
        n174 = Insert Into Array(array=dbl[][] [] ("Input Array"), new element=w622) -> (w636:dbl[][])  [unwired: 2 in]
        n175 = Number To Decimal String(number=w600) -> (decimal integer string=w625:string)  [unwired: 1 in]
        n176 = Insert Into Array(array=w636, new element=w621) -> (w635:dbl[][])  [unwired: 2 in]
        n177 = Concatenate Strings("(Vg = " ("Substring"), w627, "V, Vd = " ("Substring"), w625, "V)" ("Substring")) -> (w623:string)
        n178 = Insert Into Array(array=w635, new element=w620) -> (w634:dbl[][])  [unwired: 2 in]
        n179 = Insert Into Array(array=w634, new element=w632) -> (w631:dbl[][])  [unwired: 2 in]
        n180 = Insert Into Array(array=w631, new element=w630) -> (w597:dbl[][])  [unwired: 2 in]
        n181 = call <vilib>:"compatOverwrite.vi"("overwrite (F)"=TRUE) -> ("overwrite?"=w596:T7)
        n182 = Open/Create/Replace File(file path (use dialog)=w615, error in=w619, operation (0:open)=w596) -> (refnum out=w612:refnum<file>, error out=w613:errorcluster)  [unwired: 3 in, 1 out]
        n183 = Array To Spreadsheet String(array=w603, 3:w607) -> (spreadsheet string=w609:string)  [unwired: 1 in]
        n184 = Transpose 2D Array(2D array=w597) -> (transposed array=w629:dbl[][])
        n185 = Search and Replace String(replace all?=TRUE ("replace all? (F)"), input string=w609, search string="VgVd", replace string=w623) -> (result string=w605:string)  [unwired: 4 in, 3 out]
        n186 = Spreadsheet String To Array(format string=w607, spreadsheet string=w605, array type (2D Dbl)=w603) -> (array=w604:string[])  [unwired: 1 in]
        n187 = call "4155C Write array to file.vi"("Byte Stream File Refnum"=w612, "Header"=w604, "Data Array"=w629, "error in (no error)"=w613) -> ("dup refnum"=w610:refnum<file>, "error out"=w611:errorcluster)  [unwired: 1 in]
        n188 = Close File(refnum=w610, error in=w611) -> (error out=w598:errorcluster)  [unwired: 1 out]
      }
      frame "resample-fpp" {
        w670 = string[] ["Time /s", "Id VgVd /A", "Ig VgVd /A", "Vp1 VgVd /V", "Vp2 VgVd /V"] ("Header")
        w674 = "%d" ("format string")
        n189 = Number To Decimal String(number=w716) -> (decimal integer string=w715:string)  [unwired: 1 in]
        n190 = Fract/Exp String To Number(string=w712) -> (number=w663:dbl[])  [unwired: 3 in, 1 out]
        n191 = Concatenate Strings(w708, "-resamplefpp-" ("Substring"), w715, ".txt" ("Substring")) -> (w713:string)
        n192 = String To Path(string=w713) -> (path=w682:path)
        n193 = Index Array(array=w663, index=0 ("Index")) -> (element=w669:dbl)
        n194 = Index Array(array=w663, index=1 ("Index")) -> (element=w668:dbl)
        n195 = Number To Decimal String(number=w669) -> (decimal integer string=w692:string)  [unwired: 1 in]
        n196 = call "4155C Take Sample FPP.vi"("VISA resource name in"=w665, "error in (no error)"=w664, "Emergency Stop"=w683) -> ("Time"=w687:dbl[], "Vp1"=w697:dbl[], "VISA Resource Name out"=w667:refnum<visa-resource-name>, "Ig"=w685:dbl[], "Id"=w686:dbl[], "Vp2"=w695:dbl[], "error out"=w684:errorcluster)  [unwired: 10 in]
        n197 = Insert Into Array(array=dbl[][] [] ("Input Array"), new element=w687) -> (w701:dbl[][])  [unwired: 2 in]
        n198 = Number To Decimal String(number=w668) -> (decimal integer string=w690:string)  [unwired: 1 in]
        n199 = Insert Into Array(array=w701, new element=w686) -> (w700:dbl[][])  [unwired: 2 in]
        n200 = Concatenate Strings("(Vg = " ("Substring"), w692, "V, Vd = " ("Substring"), w690, "V)" ("Substring")) -> (w688:string)
        n201 = Insert Into Array(array=w700, new element=w685) -> (w699:dbl[][])  [unwired: 2 in]
        n202 = Insert Into Array(array=w699, new element=w697) -> (w696:dbl[][])  [unwired: 2 in]
        n203 = Insert Into Array(array=w696, new element=w695) -> (w662:dbl[][])  [unwired: 2 in]
        n204 = call <vilib>:"compatOverwrite.vi"("overwrite (F)"=TRUE) -> ("overwrite?"=w661:T7)
        n205 = Open/Create/Replace File(file path (use dialog)=w682, error in=w684, operation (0:open)=w661) -> (refnum out=w679:refnum<file>, error out=w680:errorcluster)  [unwired: 3 in, 1 out]
        n206 = Array To Spreadsheet String(array=w670, 3:w674) -> (spreadsheet string=w676:string)  [unwired: 1 in]
        n207 = Transpose 2D Array(2D array=w662) -> (transposed array=w694:dbl[][])
        n208 = Search and Replace String(replace all?=TRUE ("replace all? (F)"), input string=w676, search string="VgVd", replace string=w688) -> (result string=w672:string)  [unwired: 4 in, 3 out]
        n209 = Spreadsheet String To Array(format string=w674, spreadsheet string=w672, array type (2D Dbl)=w670) -> (array=w671:string[])  [unwired: 1 in]
        n210 = call "4155C Write array to file.vi"("Byte Stream File Refnum"=w679, "Header"=w671, "Data Array"=w694, "error in (no error)"=w680) -> ("dup refnum"=w677:refnum<file>, "error out"=w678:errorcluster)  [unwired: 1 in]
        n211 = Close File(refnum=w677, error in=w678) -> (error out=w666:errorcluster)  [unwired: 1 out]
      }
    }
    n212 = local write "Lines left to run:"(w37) -> ()
    n213 = Empty String/Path?(string/path=w37) -> (empty?=w73:bool)
    n214 = Not(x=w73) -> (.not. x?=w72:bool)
  }
